vi "TempConverter.vi"() -> ()   [LabVIEW 2018]
panel:
  out "Waveform Graph":dbl[](graph)
  out "Waveform Chart":dbl(graph)
  in  "stop":bool
  in  "Convert?":bool
  out "Thermometer":dbl(slide) scale=0.0..300.0
  in  "Temperature (F)":dbl(slide) scale=0.0..300.0
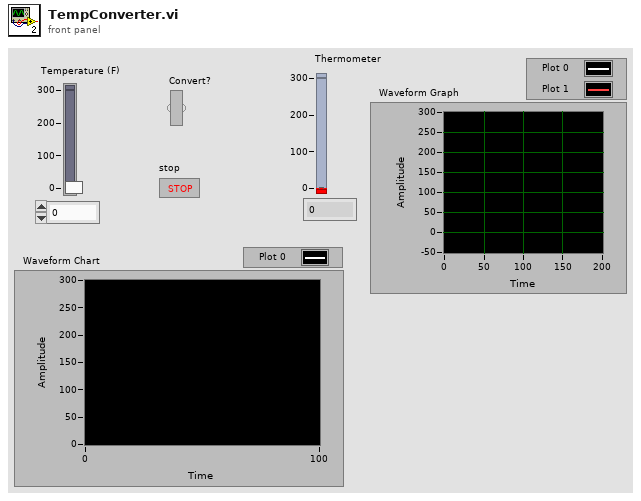
[diagram p1: front panel]
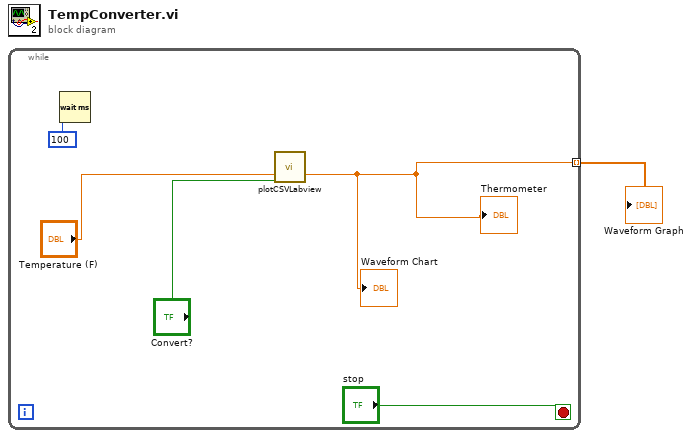
[diagram p0: block diagram]
diagram:
  n1 = while {
    tunnel: [w3] -> w1 mode=indexing
    stop <- "stop" stop-if-true
    n2 = Wait (ms)(milliseconds to wait=100) -> ()  [unwired: 1 out]
    n3 = call "plotCSVLabview.vi"("Temperature (F)"="Temperature (F)", "Boolean"="Convert?") -> ("Numeric"=w3:dbl)  [unwired: 17 in]
    "Thermometer" <- w3
    "Waveform Chart" <- w3
  }
  "Waveform Graph" <- w1
